vi "EMGCollectMain.vi"() -> ()   [LabVIEW 2015]
uses:
  <vilib>/DAQmx/write.llb/DAQmx Write (Analog DBL 1Chan 1Samp).vi
  <vilib>/DAQmx/read.llb/DAQmx Read (Analog 1D Wfm NChan NSamp).vi
  <vilib>/Analysis/baseanly.llb/Mean (DBL).vi
  <vilib>/DAQmx/create/channels.llb/DAQmx Create Channel (AI-Voltage-Basic).vi
  <vilib>/DAQmx/configure/timing.llb/DAQmx Timing (Sample Clock).vi
  <vilib>/DAQmx/create/channels.llb/DAQmx Create Channel (AO-Voltage-Basic).vi
  <vilib>/DAQmx/miscellaneous.llb/DAQmx Fill In Error Info.vi
  <vilib>/Analysis/2dsp.llb/Decimate (continuous, DBL).vi
  <vilib>/Utility/file.llb/Write Delimited Spreadsheet (I64).vi
  <resource>/objmgr/daqmx.rc
  <vilib>/Analysis/NI_AALBase.lvlib
  <vilib>/Analysis/NI_AALPro.lvlib
panel:
  in  "EMG Status":T1(radio) caption="Radio Buttons"
  in  "UsrName":string(combo) caption="User ID"
  in  "Button.Record":bool caption="TA Override"
  out "Data Path":path=path "C:/Data"
  out "RawDisp_HSR":dbl[](graph) caption="Filtered_TA"
  out "RawDisp_QCR":dbl[](graph) caption="Filtered_GL"
  out "RawDisp_HSL":dbl[](graph) caption="Filtered_QC"
  out "RawDisp_QCL":dbl[](graph) caption="Filtered_HS"
  # "HS Right"
  # "QC Right"
  # "QC Left"
  # "HS Left"
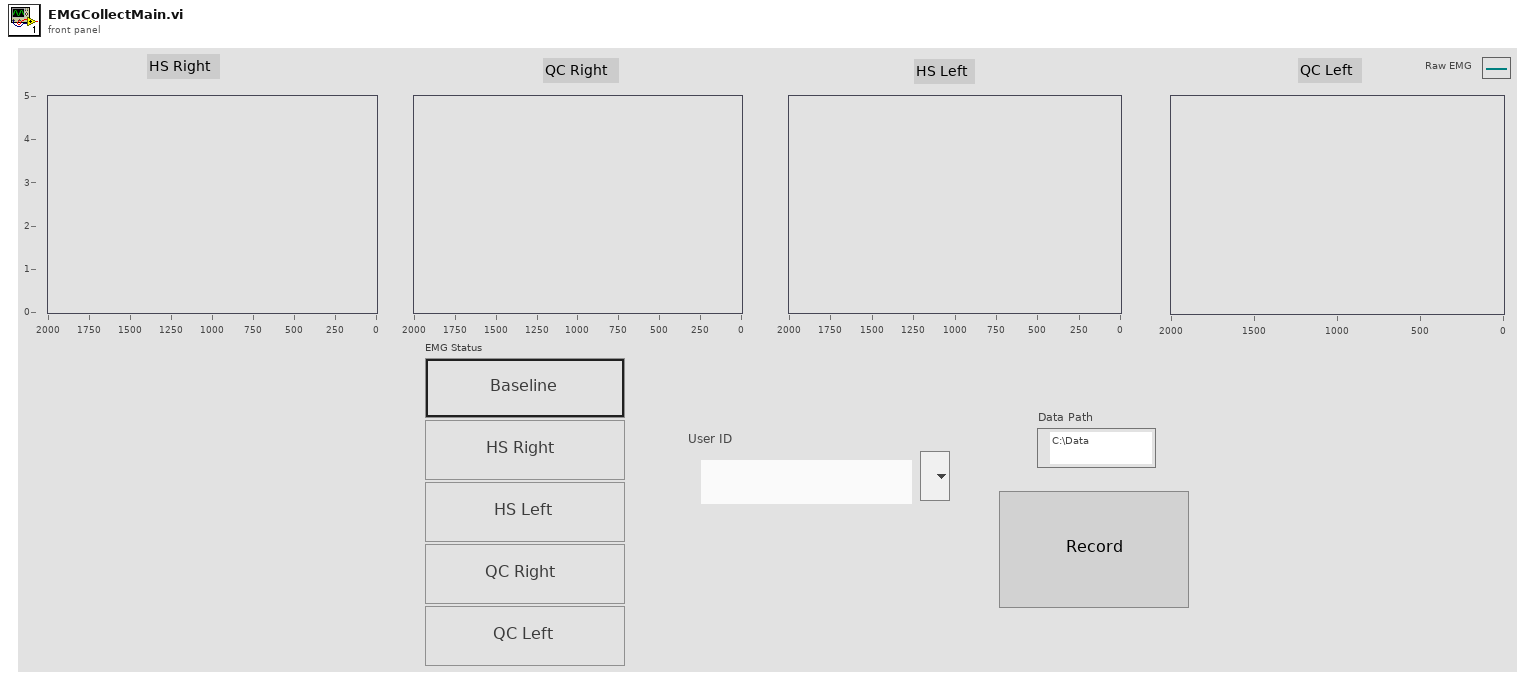
[diagram p1: front panel]
types:
  T1 = enum32{"Radio Box", "Radio Box 2", "Radio Selection 3", "Radio Selection 4", "Radio Selection 5"}
  T2 = enum16{"open", "replace", "create", "open or create", "replace or create", "replace or create with confirmation"}
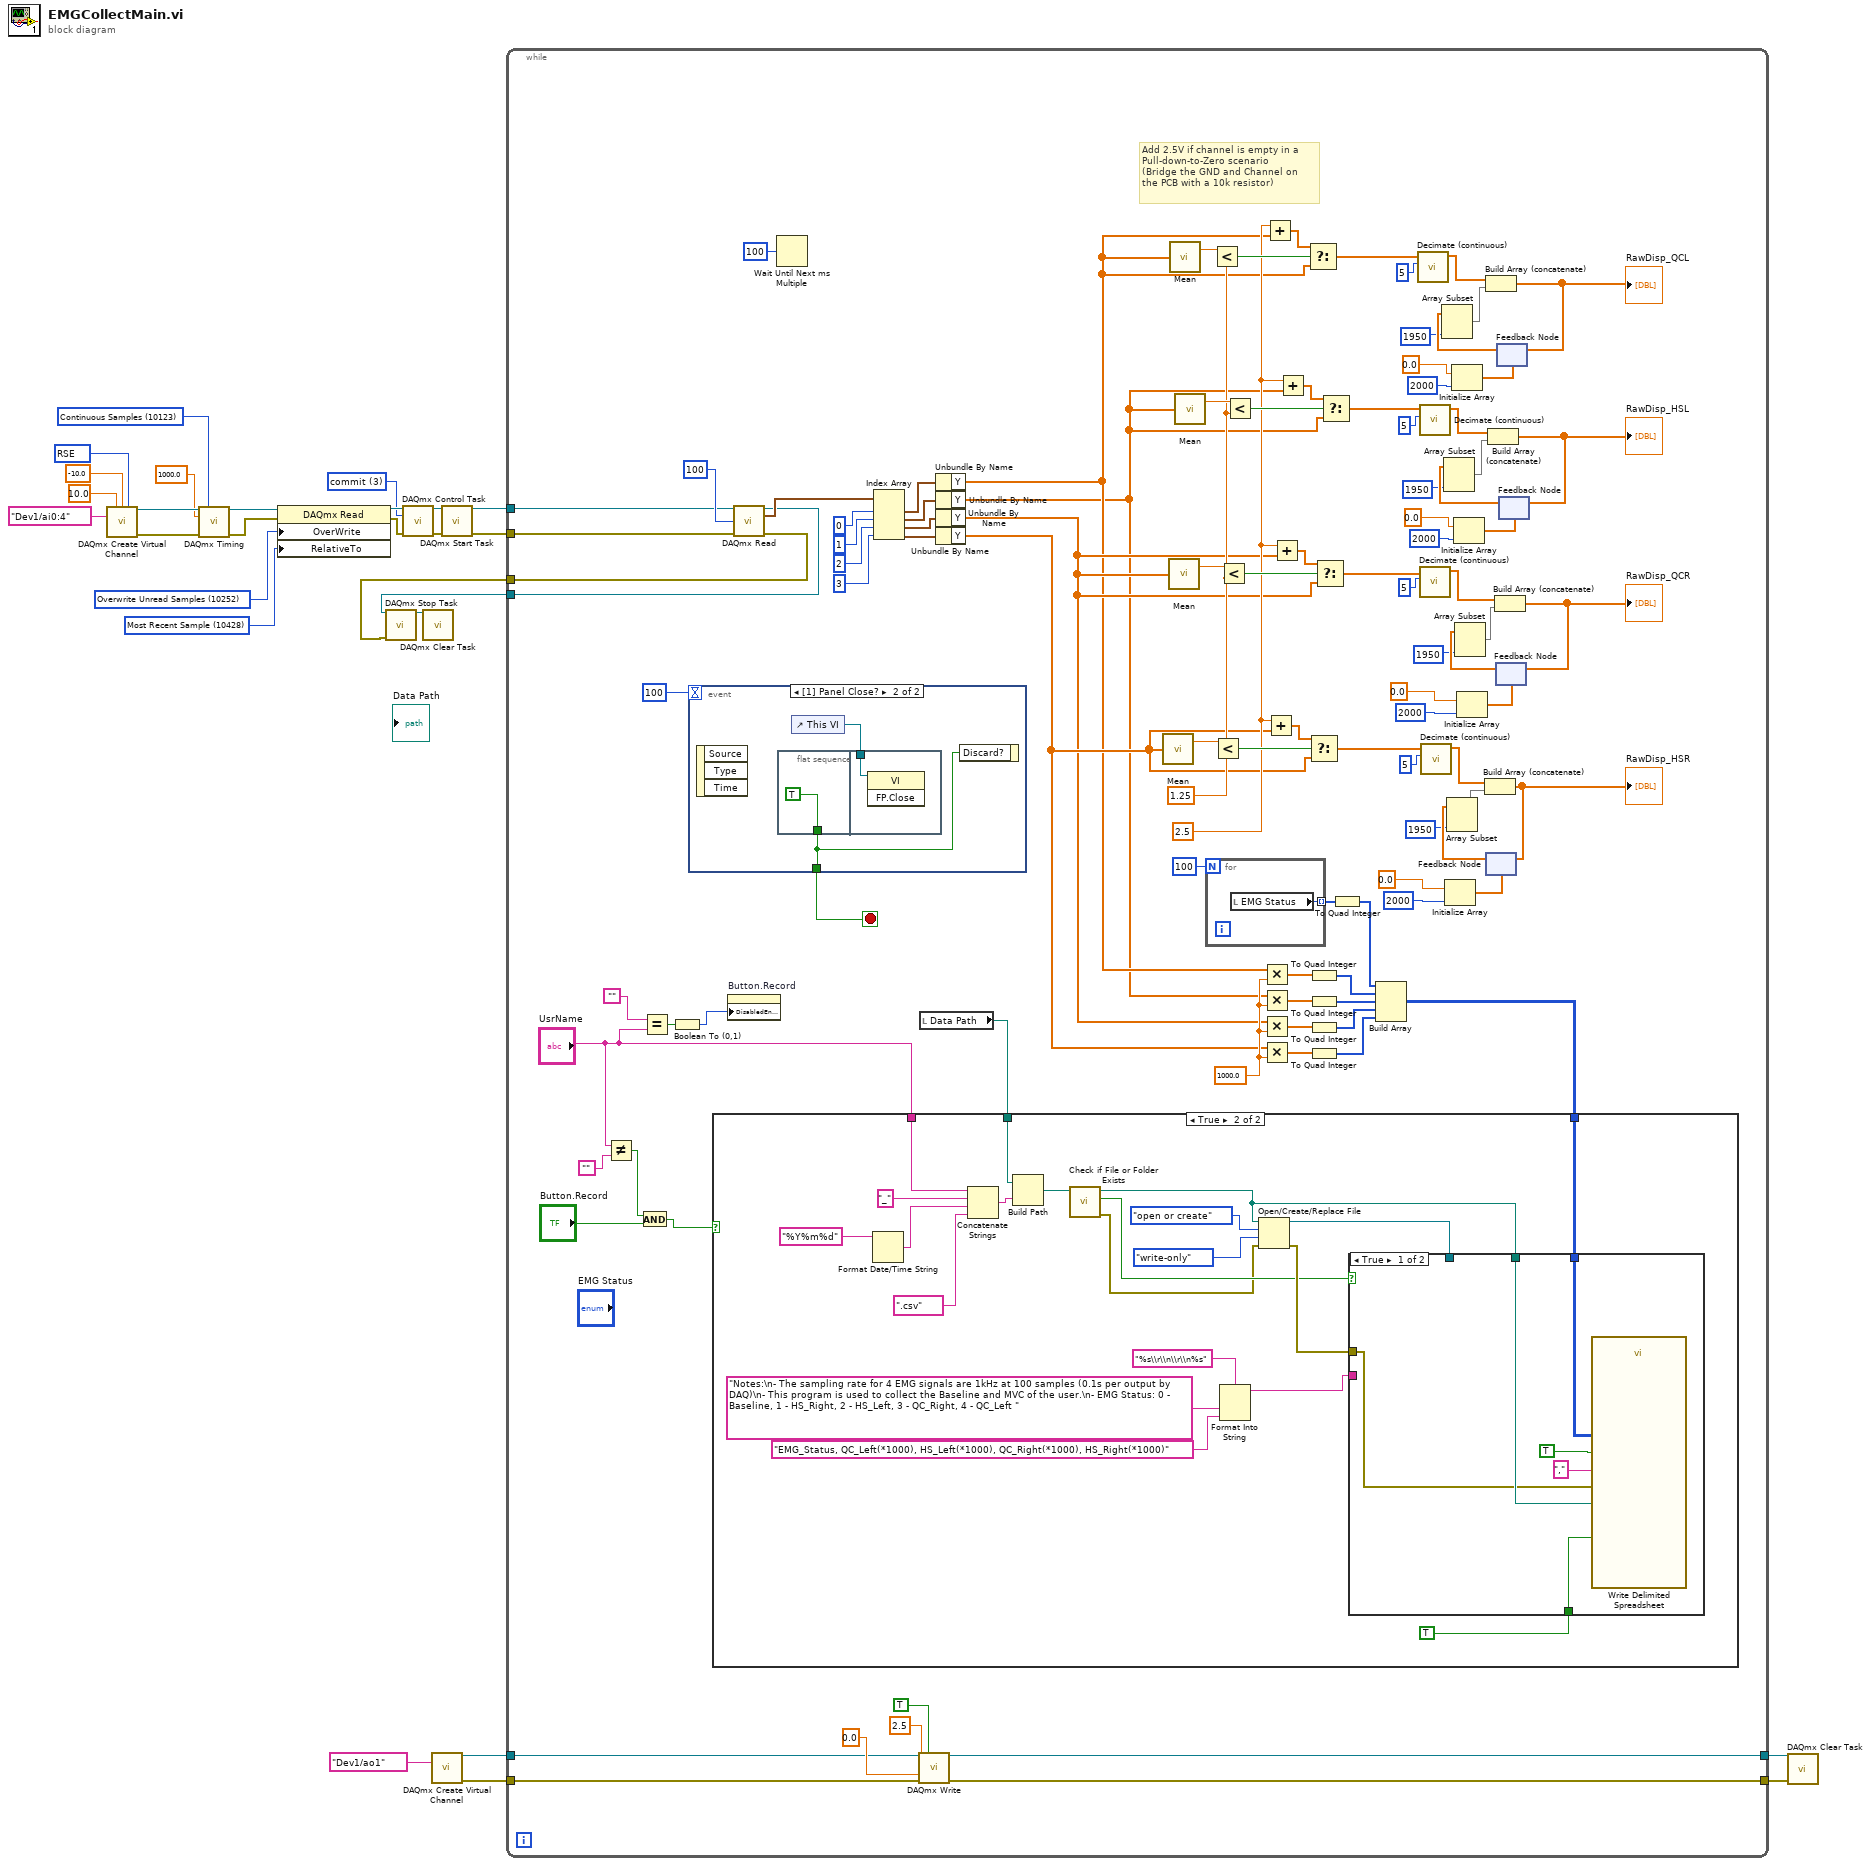
[diagram p0: block diagram]
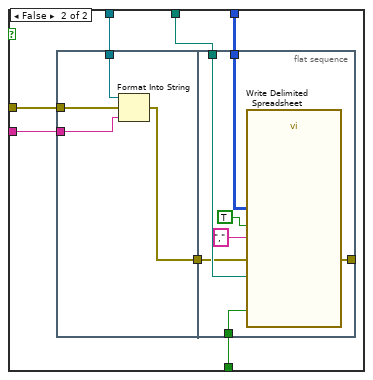
[diagram p3: hidden frame]
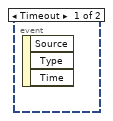
[diagram p4: hidden frame]
diagram:
  w10 = 3 items=["verify"=2, "reserve"=4, "commit"=3, "unreserve"=5, "abort"=6] ("action")
  w21 = 10083 items=["Default"=-1, "RSE"=10083, "NRSE"=10078, "Differential"=10106, "Pseudodifferential"=12529] ("input terminal configuration")
  w16 = 10428 items=["First Sample"=10424, "Current Read Position"=10425, "Reference Trigger"=10426, "First Pretrigger Sample"=10427, "Most Recent Sample"=10428] ("RelativeTo")
  w17 = 10252 items=["Overwrite Unread Samples"=10252, "Do Not Overwrite Unread Samples"=10159] ("OverWrite")
  w22 = 10123 items=["Finite Samples"=10178, "Continuous Samples"=10123, "Hardware Timed Single Point"=12522] ("sample mode")
  n1 = call-poly <vilib>:"DAQmx Create Virtual Channel.vi"("maximum value"=10.0, "minimum value"=-10.0, "input terminal configuration"=w21, "physical channels"=tag "Dev1/ai0:4") -> ("task out"=w27:refnum<k21>, "error out"=w26:errorcluster)  [unwired: 10 in]
  n2 = call-poly <vilib>:"DAQmx Timing.vi"("task/channels in"=w27, "sample mode"=w22, "rate"=1000.0, "error in"=w26) -> ("task out"=w19:refnum<k21>, "error out"=w18:errorcluster)  [unwired: 10 in]
  n3 = property class="DAQmx Read"(reference=w19, error in=w18, "OverWrite"=w17, "RelativeTo"=w16) -> (reference out=w12:refnum<k21>, error out=w11:errorcluster)
  n4 = call <vilib>:"DAQmx Control Task.vi"("task/channels in"=w12, "action"=w10, "error in"=w11) -> ("task out"=w14:refnum<k21>, "error out"=w13:errorcluster)  [unwired: 11 in]
  n5 = call-poly <vilib>:"DAQmx Create Virtual Channel.vi"("physical channels"=tag "Dev1/ao1") -> ("task out"=w2:refnum<k21>, "error out"=w1:errorcluster)  [unwired: 13 in]
  n6 = call <vilib>:"DAQmx Start Task.vi"("task/channels in"=w14, "error in"=w13) -> ("task out"=w9:refnum<k21>, "error out"=w8:errorcluster)  [unwired: 12 in]
  n7 = while {
    tunnel: w9 -> [w122]
    tunnel: w8 -> [w121]
    tunnel: [w120] -> w7
    tunnel: [w119] -> w6
    tunnel: [w58] -> w4
    tunnel: [w57] -> w3
    tunnel: w2 -> [w56]
    tunnel: w1 -> [w55]
    stop <- w131 stop-if-true
    w52 = 1000.0
    w104 = 1.25 ("x")
    w105 = 2.5 ("x")
    # "Add 2.5V if channel is empty in a \nPull-down-to-Zero scenario\n(Bridge the GND and Channel on \nthe PCB with a 10k resistor)"
    n8 = Not Equal?(x="UsrName", y="") -> (x != y?=w37:bool)
    n9 = And(x=w37, y="Button.Record") -> (x .and. y?=w36:bool)
    n10 = Equal?(x="", y="UsrName") -> (x = y?=w32:bool)
    n11 = Boolean To (0,1)(Boolean=w32) -> (0, 1=w31:i16)
    n12 = event shown="[1] Panel Close?" {
      selector: _ -> [_ _]
      dyn-events: _ -> [_ _]
      timeout: 100 -> [_ _]
      tunnel: [_ w178] -> w131
      event Timeout {
        n13 = event-data() -> ()  [unwired: 1 in, 3 out]
      }
      event Panel Close? {
        n14 = event-data() -> ()  [unwired: 1 in, 3 out]
        n15 = flat-sequence {
          tunnel: [TRUE] -> w178
          tunnel: w177 -> [w180]
          frame #0 {
          }
          frame #1 {
            n16 = invoke class="VI" method="FP.Close"(reference=w180) -> ()  [unwired: 2 in, 3 out]
          }
        }
        n17 = control-ref of="This VI"() -> (w177:refnum<vi>)
        n18 = event-data("Discard?"=w178) -> ()  [unwired: 1 in, 1 out]
      }
    }
    n19 = property on="Button.Record" class="Bool (strict)"("DisabledEnum"=w31) -> ()  [unwired: 2 in, 2 out]
    n20 = call-poly <vilib>:"DAQmx Read.vi"("task/channels in"=w122, "number of samples per channel"=100, "error in"=w121) -> ("task out"=w119:refnum<k21>, "data"=w126:waveform(dbl)[], "error out"=w120:errorcluster)  [unwired: 10 in]
    n21 = Wait Until Next ms Multiple(millisecond multiple=u32 100) -> ()  [unwired: 1 out]
    n22 = Index Array(array=w126, index #1=0 ("index"), index #2=1 ("index"), index #3=2 ("index"), index #4=3 ("index")) -> (element #1=w129:waveform(dbl), element #2=w127:waveform(dbl), element #3=w128:waveform(dbl), element #4=w118:waveform(dbl))
    n23 = call-poly <vilib>:"DAQmx Write.vi"("task/channels in"=w56, "auto start"=TRUE, "data"=2.5, "timeout"=0.0, "error in"=w55) -> ("task out"=w58:refnum<k21>, "error out"=w57:errorcluster)  [unwired: 8 in, 1 out]
    n24 = local read "Data Path"() -> (w43:path)
    n25 = Unbundle By Name(w129) -> ("Y"=w40:dbl[])
    n26 = Unbundle By Name(w127) -> ("Y"=w39:dbl[])
    n27 = Unbundle By Name(w128) -> ("Y"=w41:dbl[])
    n28 = Unbundle By Name(w118) -> ("Y"=w42:dbl[])
    n29 = call-poly <vilib>:"Mean.vi"("X"=w42) -> ("mean"=w112:dbl)  [unwired: 1 out]
    n30 = call-poly <vilib>:"Mean.vi"("X"=w41) -> ("mean"=w115:dbl)  [unwired: 1 out]
    n31 = call-poly <vilib>:"Mean.vi"("X"=w40) -> ("mean"=w106:dbl)  [unwired: 1 out]
    n32 = call-poly <vilib>:"Mean.vi"("X"=w39) -> ("mean"=w109:dbl)  [unwired: 1 out]
    n33 = for {
      N: 100 -> [_]
      tunnel: [w132] -> w29 mode=indexing
      n34 = local read "EMG Status"() -> (w132:T1)
    }
    n35 = Less?(x=w106, y=w104) -> (x < y?=w107:bool)
    n36 = Less?(x=w112, y=w104) -> (x < y?=w113:bool)
    n37 = Less?(x=w115, y=w104) -> (x < y?=w116:bool)
    n38 = Less?(x=w109, y=w104) -> (x < y?=w110:bool)
    n39 = Multiply(x=w40, y=w52) -> (x*y=w44:dbl[])
    n40 = Multiply(x=w39, y=w52) -> (x*y=w45:dbl[])
    n41 = Multiply(x=w41, y=w52) -> (x*y=w46:dbl[])
    n42 = Multiply(x=w42, y=w52) -> (x*y=w47:dbl[])
    n43 = Add(x=w105, y=w40) -> (x+y=w108:dbl[])
    n44 = Add(x=w105, y=w42) -> (x+y=w114:dbl[])
    n45 = Add(x=w105, y=w41) -> (x+y=w117:dbl[])
    n46 = Add(x=w105, y=w39) -> (x+y=w111:dbl[])
    n47 = Select(t=w108, s=w107, f=w40) -> (s? t:f=w95:dbl[])
    n48 = Select(t=w114, s=w113, f=w42) -> (s? t:f=w68:dbl[])
    n49 = To Quad Integer(1:w44) -> (0:w48:i64[])
    n50 = To Quad Integer(1:w45) -> (0:w49:i64[])
    n51 = To Quad Integer(1:w46) -> (0:w50:i64[])
    n52 = To Quad Integer(1:w47) -> (0:w51:i64[])
    n53 = Select(t=w117, s=w116, f=w41) -> (s? t:f=w77:dbl[])
    n54 = Select(t=w111, s=w110, f=w39) -> (s? t:f=w86:dbl[])
    n55 = To Quad Integer(1:w29) -> (0:w28:i64[])
    n56 = Build Array(w28, w48, w49, w50, w51) -> (w53:i64[][])
    n57 = case shown="True" w36 {
      tunnel: w53 -> [_ w153]
      tunnel: "UsrName" -> [_ w149]
      tunnel: w43 -> [_ w134]
      frame False {
      }
      frame True {
        n58 = Format Date/Time String(time format string (%c)="%Y%m%d") -> (date/time string=w146:string)  [unwired: 2 in]
        n59 = Concatenate Strings(w149, "_" ("element"), w146, ".csv") -> (w135:string)
        n60 = Build Path(base path=w134, name or relative path=w135) -> (appended path=w137:path)
        n61 = call <vilib>:"Check if File or Folder Exists.vi"("path"=w137) -> ("error out"=w140:errorcluster, "file or folder exists?"=w141:bool, "dup path"=w144:path)  [unwired: 8 in]
        n62 = Format Into String(format string="%s\\r\\n\\r\\n%s", "Notes:\n- The sampling rate for 4 EMG signals are 1kHz at 100 samples (0.1s per output by DAQ)\n- This program is used to collect the Baseline and MVC of the user.\n- EMG Status: 0 - Baseline, 1 - HS_Right, 2 - HS_Left, 3 - QC_Right, 4 - QC_Left ", "EMG_Status, QC_Left(*1000), HS_Left(*1000), QC_Right(*1000), HS_Right(*1000)" ("input 2")) -> (resulting string=w150:string)  [unwired: 2 in, 1 out]
        n63 = Open/Create/Replace File(file path (use dialog)=w144, error in=w140, operation (0:open)=T2."open or create", access (0:read/write)=enum16{"read/write", "read-only", "write-only"}."write-only") -> (refnum out=w142:refnum<file>, error out=w143:errorcluster)  [unwired: 2 in, 1 out]
        n64 = case shown="True" w141 {
          tunnel: TRUE ("transpose? (F)") -> [w157 w162]
          tunnel: w142 -> [_ w166]
          tunnel: w143 -> [w155 w165]
          tunnel: w144 -> [w156 w163]
          tunnel: w150 -> [_ w161]
          tunnel: w153 -> [w154 w160]
          frame True {
            n65 = call-poly <vilib>:"Write Delimited Spreadsheet.vi"("file path (dialog if empty)"=w156, "2D data"=w154, "append to file? (F)"=TRUE, "error in (no error)"=w155, "transpose? (F)"=w157, "delimiter (\\t)"="," ("delimiter (\\t)")) -> ()  [unwired: 8 in, 2 out]
          }
          frame False {
            n66 = flat-sequence {
              tunnel: w166 -> [w169]
              tunnel: w165 -> [w168]
              tunnel: [w170] -> w164
              tunnel: w161 -> [w167]
              tunnel: w164 -> [w172]
              tunnel: w163 -> [w175]
              tunnel: w162 -> [w173]
              tunnel: [w172] -> _
              tunnel: w160 -> [w171]
              frame #0 {
                n67 = Format Into String(initial string=w169, error in=w168, w167) -> (error out=w170:errorcluster)  [unwired: 1 in, 1 out]
              }
              frame #1 {
                n68 = call-poly <vilib>:"Write Delimited Spreadsheet.vi"("file path (dialog if empty)"=w175, "2D data"=w171, "append to file? (F)"=TRUE, "transpose? (F)"=w173, "delimiter (\\t)"="," ("delimiter (\\t)")) -> ()  [unwired: 9 in, 2 out]
              }
            }
          }
        }
      }
    }
    n69 = call-poly <vilib>:"Decimate (continuous).vi"("decimating factor"=5, "X"=w95) -> ("Decimated Array"=w97:dbl[])  [unwired: 8 in, 1 out]
    n70 = call-poly <vilib>:"Decimate (continuous).vi"("decimating factor"=5, "X"=w86) -> ("Decimated Array"=w88:dbl[])  [unwired: 8 in, 1 out]
    n71 = call-poly <vilib>:"Decimate (continuous).vi"("decimating factor"=5, "X"=w77) -> ("Decimated Array"=w79:dbl[])  [unwired: 8 in, 1 out]
    n72 = call-poly <vilib>:"Decimate (continuous).vi"("decimating factor"=5, "X"=w68) -> ("Decimated Array"=w70:dbl[])  [unwired: 8 in, 1 out]
    n73 = Initialize Array(0.0 ("element"), 2000 ("dimension size")) -> (w76:dbl[])
    n74 = Initialize Array(0.0 ("element"), 2000 ("dimension size")) -> (w103:dbl[])
    n75 = Initialize Array(0.0 ("element"), 2000 ("dimension size")) -> (w94:dbl[])
    n76 = Initialize Array(0.0 ("element"), 2000 ("dimension size")) -> (w85:dbl[])
    n77 = feedback #1(w76) -> (w73:dbl[])
    n78 = Array Subset(array=w73, length=1950 ("index")) -> (w71:dbl[])  [unwired: 1 in]
    n79 = Build Array (concatenate)(w70, w71) -> (w64:dbl[])
    "RawDisp_HSR" <- w64
    n80 = feedback-in #1(w64) -> ()
    n81 = feedback #2(w85) -> (w82:dbl[])
    n82 = Array Subset(array=w82, length=1950 ("index")) -> (w80:dbl[])  [unwired: 1 in]
    n83 = Build Array (concatenate)(w79, w80) -> (w65:dbl[])
    "RawDisp_QCR" <- w65
    n84 = feedback-in #2(w65) -> ()
    n85 = feedback #3(w103) -> (w100:dbl[])
    n86 = Array Subset(array=w100, length=1950 ("index")) -> (w98:dbl[])  [unwired: 1 in]
    n87 = Build Array (concatenate)(w97, w98) -> (w67:dbl[])
    "RawDisp_QCL" <- w67
    n88 = feedback-in #3(w67) -> ()
    n89 = feedback #4(w94) -> (w91:dbl[])
    n90 = Array Subset(array=w91, length=1950 ("index")) -> (w89:dbl[])  [unwired: 1 in]
    n91 = Build Array (concatenate)(w88, w89) -> (w66:dbl[])
    "RawDisp_HSL" <- w66
    n92 = feedback-in #4(w66) -> ()
  }
  n93 = call <vilib>:"DAQmx Stop Task.vi"("task/channels in"=w6, "error in"=w7) -> ("task out"=w15:refnum<k21>)  [unwired: 12 in, 1 out]
  n94 = call <vilib>:"DAQmx Clear Task.vi"("task in"=w15) -> ()  [unwired: 14 in, 1 out]
  n95 = call <vilib>:"DAQmx Clear Task.vi"("task in"=w4, "error in"=w3) -> ()  [unwired: 13 in, 1 out]
